vi "SVL Single Block Integration (N Ch).vi"(7 "length units":i32(ring) items=["no change"=-1, "m"=0, "mm"=2, "microns"=3, "in"=1, "mils"=5], 8 "error in (no error)":errorcluster, 9 "known conditions":T1[](array[typedef])=[{"condition type"=enum."Initial Value", "known value"=nan}], 11 "scaled signals [EU]":waveform(dbl)[](array[waveform])) -> (0 "error out":errorcluster, 2 "unit labels":string[](array[string]), 3 "integrated signal":waveform(dbl)[](array[waveform]))   [LabVIEW 2017, in "SoundVib_Integration.lvlib"]
doc: "Converts acceleration to velocity or displacement using a time-domain waveform as the input. Wire data to the <B>scaled signal [EU]</B> input to determine the polymorphic instance to use or manually select the instance.\n\nPerforms single integration on a single block of data. Use this VI to numerically integrate a single block of data. Use the known condition input to correct the integrated signal for that known condition. The <B>condition type</B> value of the <B>known condition</B> input determines how the intergrated signal is adjusted, and the <B>known value</B> determines by how much it is adjusted. <B>condition type</B> can be <B>Initial Value</B>, <B>Mean Value</B>, or <B>Final Value</B>. Using <B>Initial Value</B> will offset the integrated signal so that the first value is eqaul to the known value. Using <B>Mean Value</B> will offset the integrated signal so that its mean is eqaul to the known value. And finally, using <B>Final Value</B> will offset the integrated signal so that its last value is eqaul to the known value. If <B>known value</B> is set to NaN, no adjustment will be performed (this is the default if unwired)."
uses:
  <vilib>/addons/Sound and Vibration/svt_Integration/SoundVib_Integration.lvlib
  <vilib>/addons/_NISVFA/_Shared subVIs/Controls/svc_Integration Known Condition.ctl
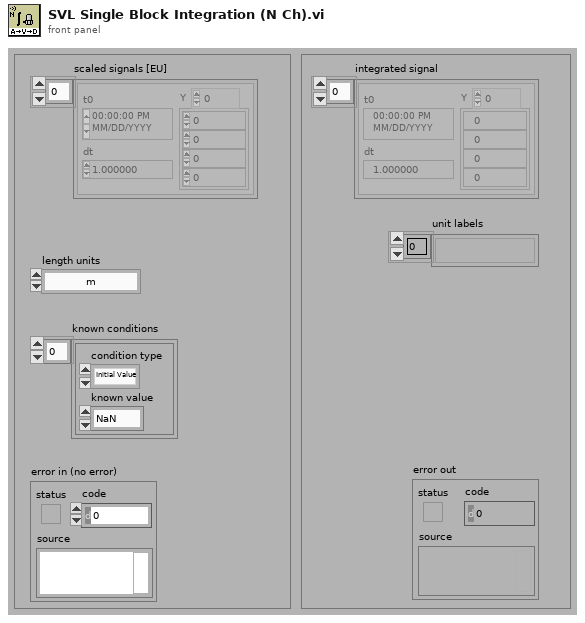
[diagram p1: front panel]
types:
  T1 = typedef "svc_Integration Known Condition.ctl" = cluster{"condition type":enum16{"Initial Value", "Mean Value", "Final Value"}, "known value":dbl}
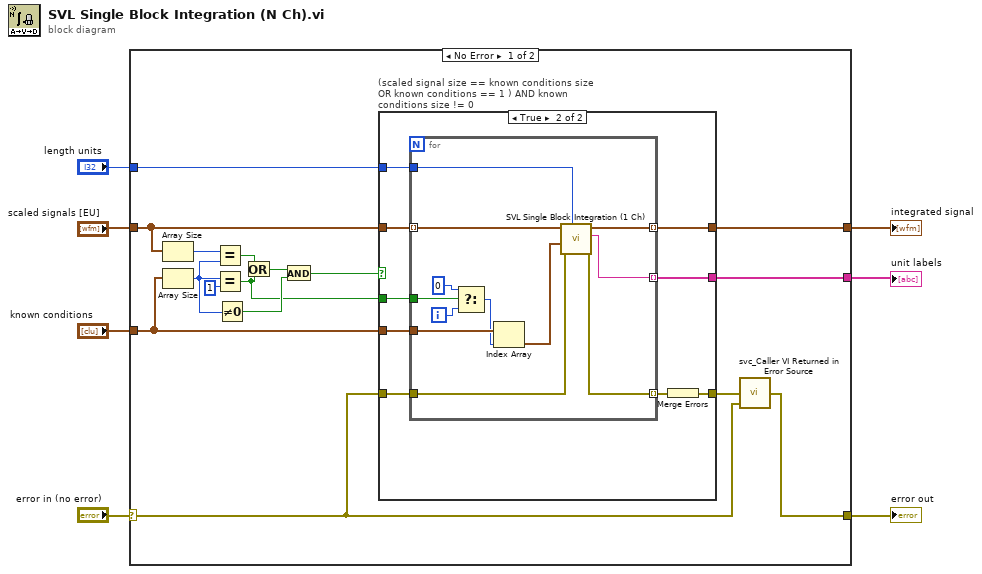
[diagram p0: block diagram]
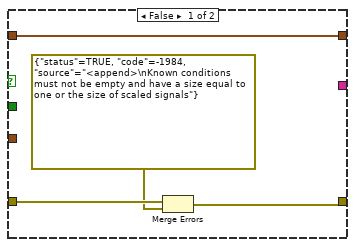
[diagram p2: hidden frame]
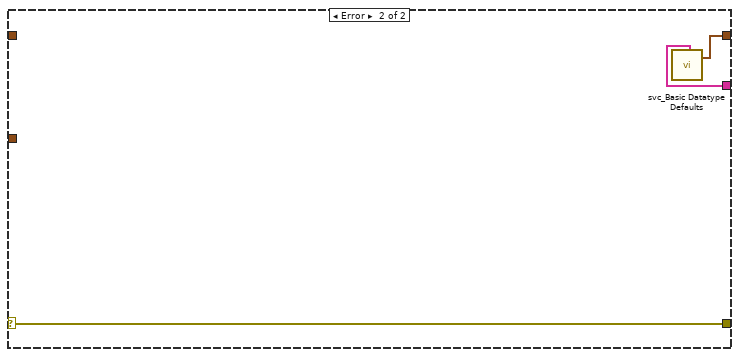
[diagram p3: hidden frame]
diagram:
  n1 = case shown="No Error" "error in (no error)" {
    selector: "error in (no error)" -> [w11 w51]
    tunnel: "scaled signals [EU]" -> [w19 _]
    tunnel: [w21 w49] -> w4
    tunnel: [w23 w51] -> w1
    tunnel: [w8 w50] -> w2
    tunnel: "length units" -> [w22 _]
    tunnel: "known conditions" -> [w20 _]
    frame No Error {
      n2 = Array Size(array=w19) -> (size(s)=w18:i32)
      n3 = Array Size(array=w20) -> (size(s)=w15:i32)
      n4 = Equal?(x=w18, y=w15) -> (x = y?=w16:bool)
      n5 = Equal?(x=w15, y=1) -> (x = y?=w9:bool)
      n6 = Not Equal To 0?(x=w15) -> (x != 0?=w13:bool)
      n7 = Or(x=w16, y=w9) -> (x .or. y?=w14:bool)
      n8 = And(x=w14, y=w13) -> (x .and. y?=w12:bool)
      n9 = case "(scaled signal size == known conditions size OR known conditions == 1 ) AND known conditions size != 0" shown="True" w12 {
        tunnel: w22 -> [_ w36]
        tunnel: [w27 w35] -> w21
        tunnel: w20 -> [_ w34]
        tunnel: w19 -> [w27 w33]
        tunnel: w11 -> [w26 w31]
        tunnel: [w25 w32] -> w10
        tunnel: w9 -> [_ w30]
        tunnel: [_ w28] -> w8
        frame False {
          n10 = Merge Errors(w26, errorcluster {"status"=TRUE, "code"=-1984, "source"="<append>\nKnown conditions must not be empty and have a size equal to one or the size of scaled signals"} ("error in")) -> (w25:errorcluster)
        }
        frame True {
          n11 = for {
            tunnel: w33 -> [w43] mode=indexing
            tunnel: w36 -> [w38]
            tunnel: [w42] -> w35 mode=indexing
            tunnel: w34 -> [w48]
            tunnel: w31 -> [w40]
            tunnel: w30 -> [w47]
            tunnel: [w39] -> w29 mode=indexing
            tunnel: [w37] -> w28 mode=indexing
            i -> [w46]
            n12 = Select(t=0, s=w47, f=w46) -> (s? t:f=w44:i32)
            n13 = Index Array(array=w48, index=w44) -> (element=w41:T1)
            n14 = call <vilib>:"SVL Single Block Integration (1 Ch).vi"("length units"=w38, "error in (no error)"=w40, "known condition"=w41, "scaled signal [EU]"=w43) -> ("error out"=w39:errorcluster, "unit label"=w37:string, "integrated signal [EU*s]"=w42:waveform(dbl))  [unwired: 5 in]
          }
          n15 = Merge Errors(w29) -> (w32:errorcluster)
        }
      }
      n16 = call <vilib>:"svc_Caller VI Returned in Error Source.vi"("warning input to caller"=w11, "error in (no error)"=w10) -> ("error out"=w23:errorcluster)  [unwired: 3 in]
    }
    frame Error {
      n17 = call <vilib>:"svc_Basic Datatype Defaults.vi"() -> ("empty array of strings"=w50:string[], "empty array of waveforms"=w49:waveform(dbl)[])  [unwired: 7 in, 11 out]
    }
  }
  "error out" <- w1
  "integrated signal" <- w4
  "unit labels" <- w2
